vi "LJM logger default scaling equations to input vars.vi"(1 "Default Scaling Equations":string[](array[string])) -> (0 "Scaling Equation Input Variables":string[](array[string]))   [LabVIEW 2026]
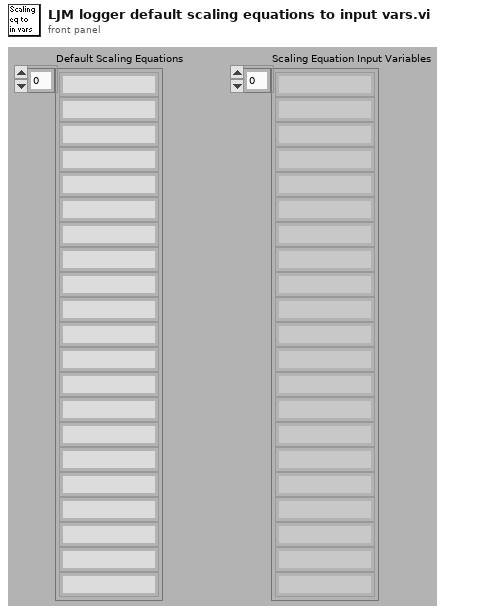
[diagram p1: front panel]
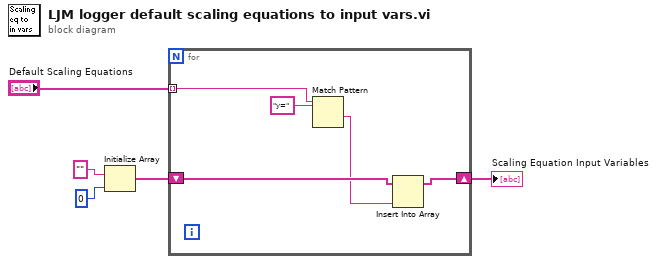
[diagram p0: block diagram]
diagram:
  n1 = Initialize Array("", 0 ("dimension size")) -> (w2:string[])
  n2 = for {
    tunnel: "Default Scaling Equations" -> [w10] mode=indexing
    shift-right: [w7] -> w1
    shift-left: w2 -> [w8]
    n3 = Match Pattern(string=w10, regular expression="y=") -> (after substring=w6:string)  [unwired: 1 in, 3 out]
    n4 = Insert Into Array(array=w8, new element=w6) -> (w7:string[])  [unwired: 1 in]
  }
  "Scaling Equation Input Variables" <- w1
